vi "controlAmplitude.vi"(7 "Set":bool, 8 "error in":errorcluster, 9 "amplitude [V] in":dbl, 10 "axis in":u8, 11 "connection ID":refnum<k5>) -> (0 "error out":errorcluster, 1 "amplitude [V] out":dbl, 2 "axis out":u8, 3 "connection ID":refnum<k5>)   [LabVIEW 2016]
panel:
  in  "Set Command":string="com.attocube.amc.control.setControlAmplitude"
  in  "Get Command":string="com.attocube.amc.control.getControlAmplitude"
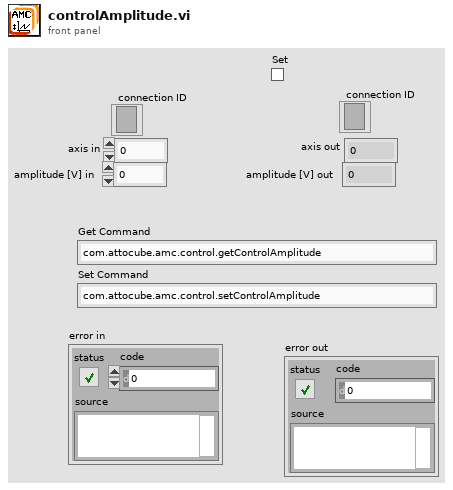
[diagram p1: front panel]
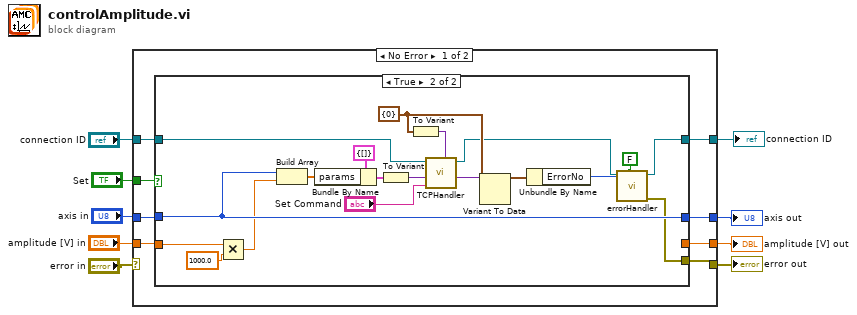
[diagram p0: block diagram]
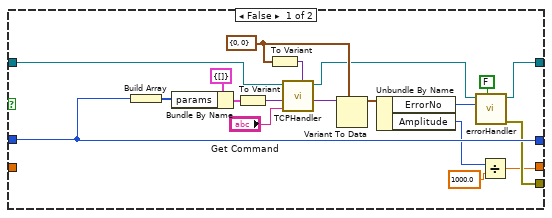
[diagram p2: hidden frame]
diagram:
  n1 = case shown="No Error" "error in" {
    selector: "error in" -> [_ w59]
    tunnel: "axis in" -> [w17 w58]
    tunnel: [w13 w59] -> w8
    tunnel: [w16 w58] -> w7
    tunnel: "amplitude [V] in" -> [w11 w56]
    tunnel: [w14 w56] -> w2
    tunnel: "Set" -> [w10 _]
    tunnel: [w12 w57] -> w5
    tunnel: "connection ID" -> [w15 w57]
    frame No Error {
      n2 = case shown="True" w10 {
        tunnel: [w18 w37] -> w12
        tunnel: w15 -> [w26 w50]
        tunnel: w17 -> [w28 w48]
        tunnel: [w28 w48] -> w16
        tunnel: [w20 _] -> w14
        tunnel: [w27 w45] -> w13
        tunnel: w11 -> [_ w39]
        frame False {
          w24 = cluster{"ErrorNo":i16, "Amplitude":i64} {"ErrorNo"=0, "Amplitude"=0} ("input cluster")
          n3 = Build Array(w28) -> (w32:u8[])
          n4 = Bundle By Name(cluster=cluster{"params":i16[]} {"params"=[]} ("input cluster"), "params"=w32) -> (w33:cluster{"params":i16[]})
          n5 = To Variant(anything=w33) -> (Variant=w34:variant)
          n6 = To Variant(anything=w24) -> (Variant=w25:variant)
          n7 = call "TCPHandler.vi"("result Types"=w25, "method"="Get Command", "params"=w34, "connection ID"=w26) -> ("result"=w30:variant, "connection ID"=w19:refnum<k5>)  [unwired: 5 in, 1 out]
          n8 = Variant To Data(type=w24, Variant=w30) -> (data=w35:cluster{"ErrorNo":i16, "Amplitude":i64})  [unwired: 1 in, 1 out]
          n9 = Unbundle By Name(w35) -> ("ErrorNo"=w36:i16, "Amplitude"=w21:i64)
          n10 = call "errorHandler.vi"("show popup"=FALSE, "error number"=w36, "connection ID"=w19) -> ("error out"=w27:errorcluster, "connection ID"=w18:refnum<k5>)  [unwired: 7 in]
          n11 = Divide(x=w21, y=1000.0) -> (x/y=w20:dbl)
        }
        frame True {
          w43 = cluster{"ErrorNo":i16} {"ErrorNo"=0} ("input cluster")
          n12 = Multiply(x=w39, y=1000.0) -> (x*y=w40:dbl)
          n13 = Build Array(w48, w40) -> (w52:dbl[])
          n14 = Bundle By Name(cluster=cluster{"params":dbl[]} {"params"=[]} ("input cluster"), "params"=w52) -> (w51:cluster{"params":dbl[]})
          n15 = To Variant(anything=w51) -> (Variant=w49:variant)
          n16 = To Variant(anything=w43) -> (Variant=w44:variant)
          n17 = call "TCPHandler.vi"("result Types"=w44, "method"="Set Command", "params"=w49, "connection ID"=w50) -> ("result"=w54:variant, "connection ID"=w38:refnum<k5>)  [unwired: 5 in, 1 out]
          n18 = Variant To Data(type=w43, Variant=w54) -> (data=w47:cluster{"ErrorNo":i16})  [unwired: 1 in, 1 out]
          n19 = Unbundle By Name(w47) -> ("ErrorNo"=w46:i16)
          n20 = call "errorHandler.vi"("show popup"=FALSE, "error number"=w46, "connection ID"=w38) -> ("error out"=w45:errorcluster, "connection ID"=w37:refnum<k5>)  [unwired: 7 in]
        }
      }
    }
    frame Error {
    }
  }
  "error out" <- w8
  "axis out" <- w7
  "amplitude [V] out" <- w2
  "connection ID" <- w5
